vi "Initialize Worktable.vi"(8 "error in":errorcluster, 10 "Project Path":path, 11 "Gantry in":refnum<class "Gantry.lvclass">) -> (0 "error out":errorcluster, 3 "Gantry out":refnum<class "Gantry.lvclass">)   [LabVIEW 2022 SP3, in "Gantry.lvclass"]
uses:
  Gantry.lvclass
  Gantry.lvclass/Gantry.ctl
  FlexWorktable/FlexWorktable.lvclass
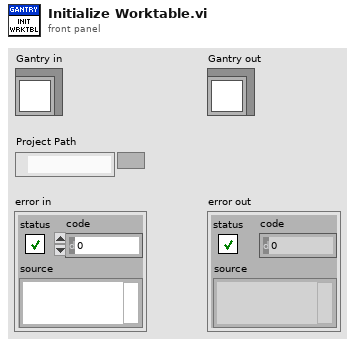
[diagram p1: front panel]
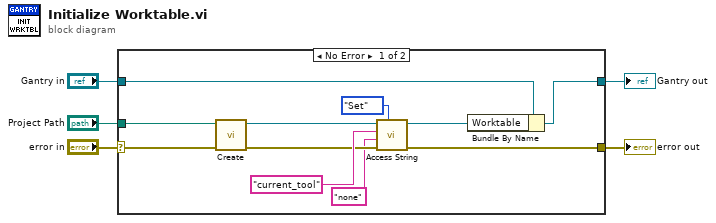
[diagram p0: block diagram]
diagram:
  n1 = case shown="No Error" "error in" {
    selector: "error in" -> [w14 w18]
    tunnel: [w7 w18] -> w4
    tunnel: [w15 w17] -> w2
    tunnel: "Gantry in" -> [w16 w17]
    tunnel: "Project Path" -> [w6 _]
    frame No Error {
      n2 = call "Create.vi"("error in (no error)"=w14, "Project Path"=w6) -> ("error out"=w11:errorcluster, "FlexWorktable out"=w13:refnum<class "FlexWorktable.lvclass">)  [unwired: 8 in]
      n3 = call-dynamic "Access String.vi"("Get/Set"=enum16{"Get", "Set"}."Set", "error in (no error)"=w11, "Value in"="none", "Key"="current_tool", "FlexWorktable in"=w13) -> ("error out"=w7:errorcluster, "FlexWorktable out"=w9:refnum<class "FlexWorktable.lvclass">)  [unwired: 4 in, 1 out]
      n4 = Bundle By Name(cluster=w16, "Worktable"=w9) -> (w15:refnum<class "Gantry.lvclass">)
    }
    frame Error {
    }
  }
  "error out" <- w4
  "Gantry out" <- w2
